vi "Disable All.vi"(8 "error in":errorcluster) -> (0 "error out":errorcluster)   [LabVIEW 2024, in "Logging.lvlib" / "Registry.lvlib"]
uses:
  Registry.lvlib
  Registry Actions.ctl
panel:
  # "Connector Pane"
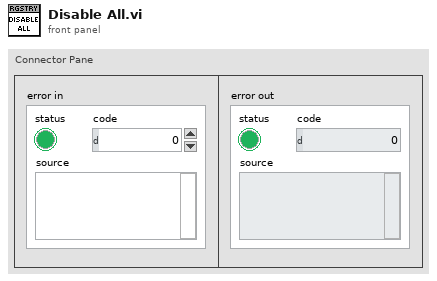
[diagram p1: front panel]
types:
  T1 = typedef "Logging.lvlib/Registry.lvlib/Registry Actions.ctl" = enum16{"Register", "Log", "Enable", "Enable All", "Disable", "Disable All", "List", "Unregister", "Unregister All"}
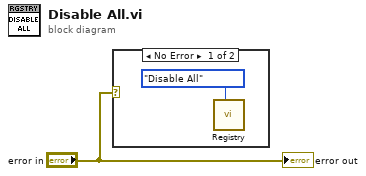
[diagram p0: block diagram]
diagram:
  n1 = case shown="No Error" "error in" {
    frame No Error {
      n2 = call "Registry.vi"("action"=Registry_Actions."Disable All") -> ()  [unwired: 9 in, 2 out]
    }
    frame Error {
    }
  }
  "error out" <- "error in"
